vi "String - Create comma seperated String.vi"(9 "C":string, 10 "B":string, 11 "A":string) -> (3 "A, B , C (auto comma)":string)   [LabVIEW 2013]
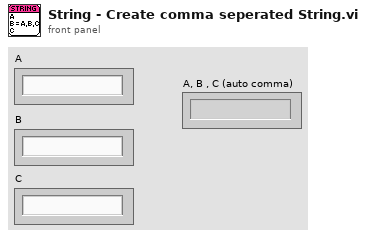
[diagram p1: front panel]
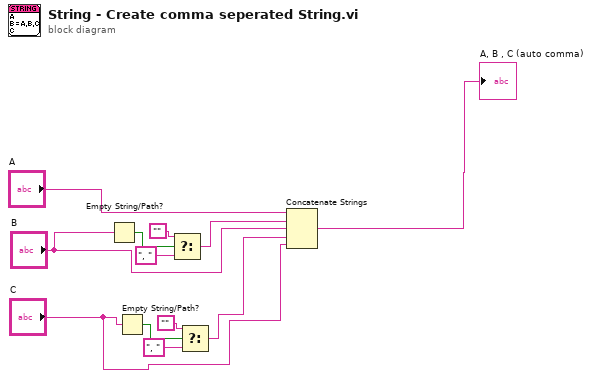
[diagram p0: block diagram]
diagram:
  n1 = Empty String/Path?(string/path="B") -> (empty?=w7:bool)
  n2 = Empty String/Path?(string/path="C") -> (empty?=w5:bool)
  n3 = Select(t="", s=w7, f=", ") -> (s? t:f=w10:string)
  n4 = Select(t="", s=w5, f=", ") -> (s? t:f=w2:string)
  n5 = Concatenate Strings("A", w10, "B", w2, "C") -> (→"A, B , C (auto comma)":string)
